vi "Intellirupter_sensor2.vi"() -> ()   [LabVIEW 2016]
uses:
  <vilib>/rvi/Emulation/niFpgaGetClockAttributes.vi
  <vilib>/rvi/Emulation/niFpgaSctlEmulationGetInTimedLoop.vi
  <vilib>/rvi/Emulation/niFpgaEmulationReportErrorSimple.vi
  <vilib>/rvi/eio/common/nirviEmuTemplateMethod_errors.vi
  <vilib>/rvi/Emulation/niFpgaCriticalErrorInLSC.vi
  <vilib>/eio/EIONode/EIONode.xnode
panel:
  out "I8 B":fxp<+/-,26,5>
  out "I8 A":fxp<+/-,26,5>
  out "V8R CA":fxp<+/-,26,5>
  out "V8R BC":fxp<+/-,26,5>
  out "V8R AB":fxp<+/-,26,5>
  out "V5R CA":fxp<+/-,26,5>
  out "V5R BC":fxp<+/-,26,5>
  out "V5R AB":fxp<+/-,26,5>
  out "I5 B":fxp<+/-,26,5>
  out "I5 A":fxp<+/-,26,5>
  out "V5L CA":fxp<+/-,26,5>
  out "V5L BC":fxp<+/-,26,5>
  out "V5L AB":fxp<+/-,26,5>
  out "V4L CA":fxp<+/-,26,5>
  out "V4L BC":fxp<+/-,26,5>
  out "V4L AB":fxp<+/-,26,5>
  out "I4 C":fxp<+/-,26,5>
  out "I4 B":fxp<+/-,26,5>
  out "I4 A":fxp<+/-,26,5>
  out "V4R CA":fxp<+/-,26,5>
  out "V4R BC":fxp<+/-,26,5>
  out "V4R AB":fxp<+/-,26,5>
  out "V2L CA":fxp<+/-,26,5>
  out "V2L BC":fxp<+/-,26,5>
  out "V2L AB":fxp<+/-,26,5>
  out "I2 C":fxp<+/-,26,5>
  out "I5 C":fxp<+/-,26,5>
  out "I2 B":fxp<+/-,26,5>
  out "I2 A":fxp<+/-,26,5>
  out "V2R CA":fxp<+/-,26,5>
  out "V2R BC":fxp<+/-,26,5>
  out "V2R AB":fxp<+/-,26,5>
  out "V7R CA":fxp<+/-,26,5>
  out "V7R BC":fxp<+/-,26,5>
  out "V7R AB":fxp<+/-,26,5>
  out "I8 C":fxp<+/-,26,5>
  out "V8L CA":fxp<+/-,26,5>
  out "V8L BC":fxp<+/-,26,5>
  out "V8L AB":fxp<+/-,26,5>
  out "I7 C":fxp<+/-,26,5>
  out "I7 B":fxp<+/-,26,5>
  out "I7 A":fxp<+/-,26,5>
  out "V7L CA":fxp<+/-,26,5>
  out "V7L BC":fxp<+/-,26,5>
  out "V7L AB":fxp<+/-,26,5>
  out "V6R CA":fxp<+/-,26,5>
  out "V6R BC":fxp<+/-,26,5>
  out "V6R AB":fxp<+/-,26,5>
  out "I6 C":fxp<+/-,26,5>
  out "I6 B":fxp<+/-,26,5>
  out "I6 A":fxp<+/-,26,5>
  out "V6L CA":fxp<+/-,26,5>
  out "V6L BC":fxp<+/-,26,5>
  out "V6L AB":fxp<+/-,26,5>
  out "V3L CA":fxp<+/-,26,5>
  out "V3L BC":fxp<+/-,26,5>
  out "V3L AB":fxp<+/-,26,5>
  out "I3 C":fxp<+/-,26,5>
  out "I3 B":fxp<+/-,26,5>
  out "I3 A":fxp<+/-,26,5>
  out "V3R CA":fxp<+/-,26,5>
  out "V3R BC":fxp<+/-,26,5>
  out "V3R AB":fxp<+/-,26,5>
  out "V1L CA":fxp<+/-,26,5>
  out "V1L BC":fxp<+/-,26,5>
  out "V1L AB":fxp<+/-,26,5>
  out "I1 C":fxp<+/-,26,5>
  out "I1 B":fxp<+/-,26,5>
  out "I1 A":fxp<+/-,26,5>
  out "V1R CA":fxp<+/-,12,5>
  out "V1R BC":fxp<+/-,26,5>
  out "V1R AB":fxp<+/-,26,5>
  in  "Count(ticks)":u32=100
  in  "Relay8":bool
  in  "Relay7":bool
  in  "Relay6":bool
  in  "Relay5":bool
  in  "Relay4":bool
  in  "Relay3":bool
  in  "Relay2":bool
  in  "Relay1":bool
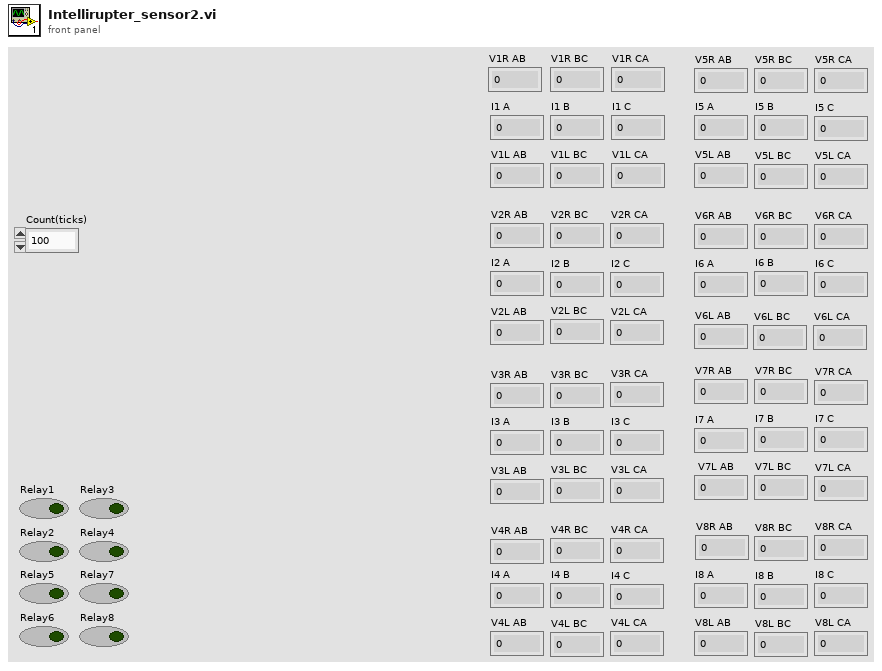
[diagram p1: front panel]
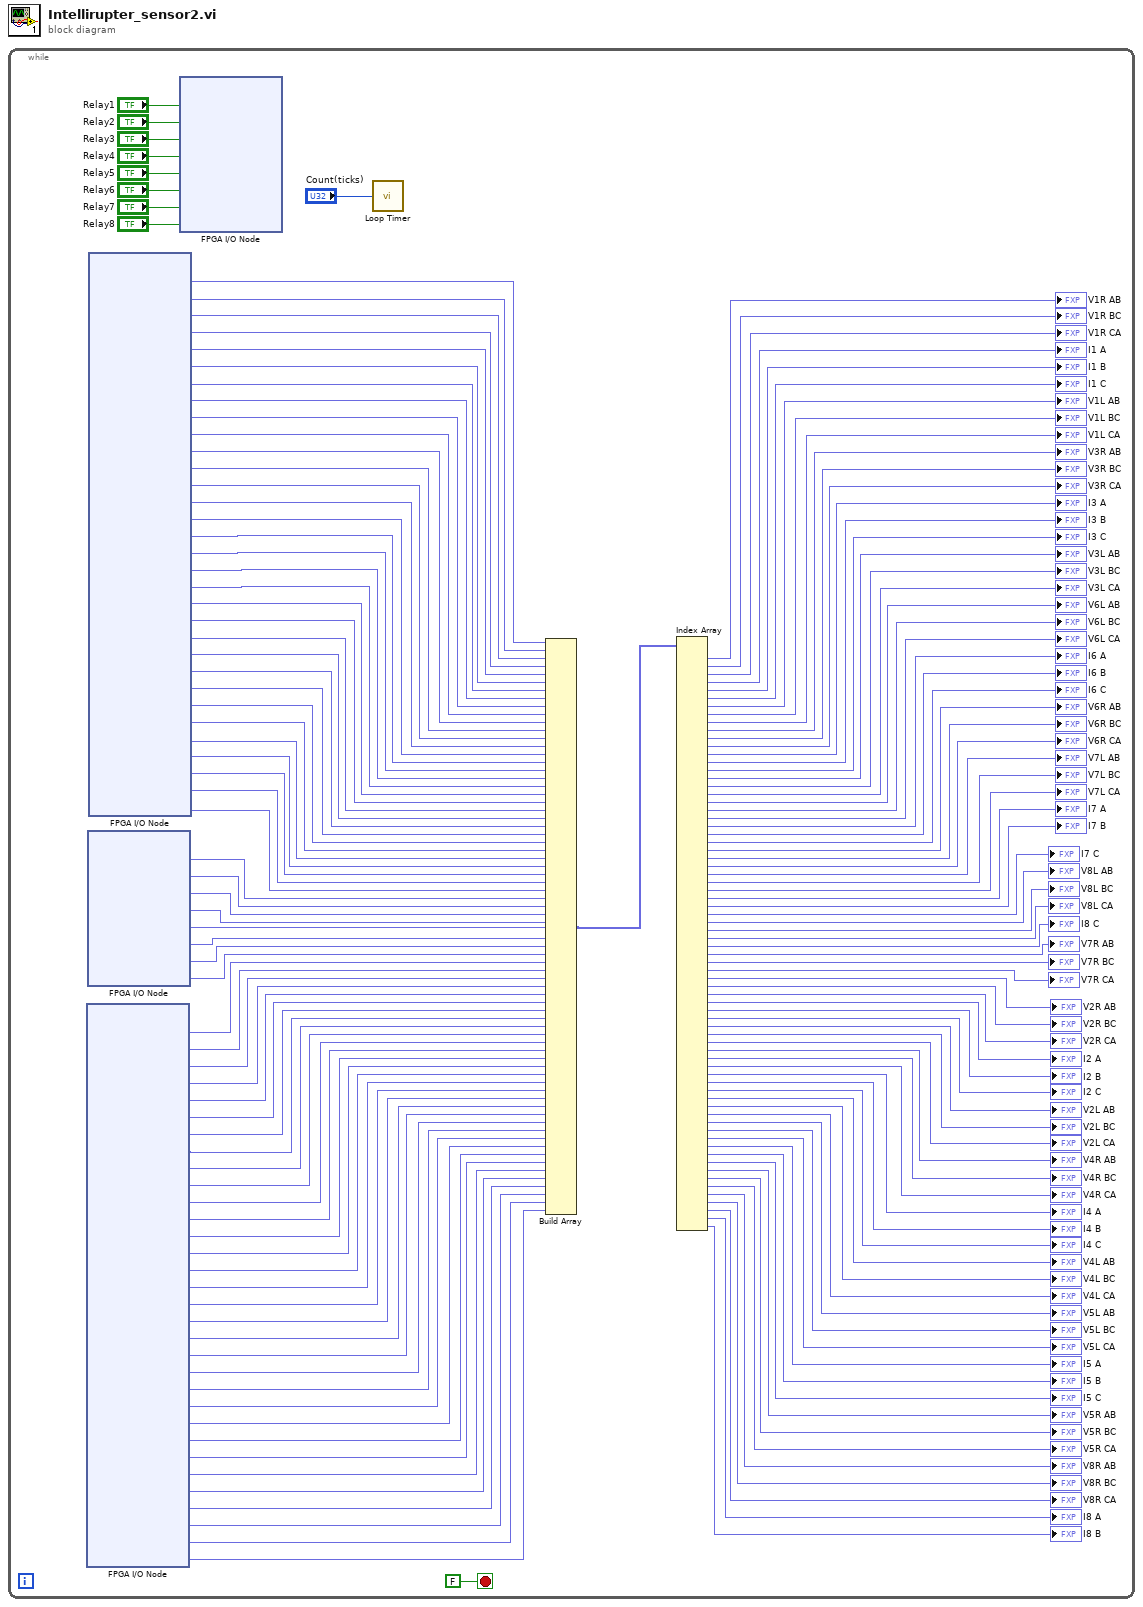
[diagram p0: block diagram]
diagram:
  n1 = while {
    stop <- FALSE stop-if-true
    n2 = xnode "FPGA I/O Node"() -> ("Mod7/AI0"=w114:fxp<+/-,26,5>, "Mod7/AI1"=w104:fxp<+/-,26,5>, "Mod7/AI2"=w103:fxp<+/-,26,5>, "Mod7/AI3"=w102:fxp<+/-,26,5>, "Mod7/AI4"=w101:fxp<+/-,26,5>, "Mod7/AI5"=w100:fxp<+/-,26,5>, "Mod7/AI6"=w99:fxp<+/-,26,5>, "Mod7/AI7"=w98:fxp<+/-,26,5>, "Mod7/AI8"=w97:fxp<+/-,26,5>, "Mod7/AI9"=w96:fxp<+/-,26,5>, "Mod7/AI10"=w95:fxp<+/-,26,5>, "Mod7/AI11"=w94:fxp<+/-,26,5>, "Mod7/AI12"=w93:fxp<+/-,26,5>, "Mod7/AI13"=w92:fxp<+/-,26,5>, "Mod7/AI14"=w74:fxp<+/-,26,5>, "Mod7/AI15"=w75:fxp<+/-,26,5>, "Mod7/AI16"=w76:fxp<+/-,26,5>, "Mod7/AI17"=w77:fxp<+/-,26,5>, "Mod7/AI18"=w78:fxp<+/-,26,5>, "Mod7/AI19"=w79:fxp<+/-,26,5>, "Mod7/AI20"=w80:fxp<+/-,26,5>, "Mod7/AI21"=w81:fxp<+/-,26,5>, "Mod7/AI22"=w82:fxp<+/-,26,5>, "Mod7/AI23"=w83:fxp<+/-,26,5>, "Mod7/AI24"=w84:fxp<+/-,26,5>, "Mod7/AI25"=w85:fxp<+/-,26,5>, "Mod7/AI26"=w86:fxp<+/-,26,5>, "Mod7/AI27"=w87:fxp<+/-,26,5>, "Mod7/AI28"=w88:fxp<+/-,26,5>, "Mod7/AI29"=w89:fxp<+/-,26,5>, "Mod7/AI30"=w90:fxp<+/-,26,5>, "Mod7/AI31"=w91:fxp<+/-,26,5>)  [unwired: 32 in, 32 out]
    n3 = xnode "FPGA I/O Node"() -> ("Mod5/AI20"=w122:fxp<+/-,26,5>, "Mod5/AI1"=w121:fxp<+/-,26,5>, "Mod5/AI2"=w120:fxp<+/-,26,5>, "Mod5/AI3"=w119:fxp<+/-,26,5>, "Mod5/AI0"=w118:fxp<+/-,26,5>, "Mod5/AI21"=w117:fxp<+/-,26,5>, "Mod5/AI22"=w116:fxp<+/-,26,5>, "Mod5/AI23"=w115:fxp<+/-,26,5>)  [unwired: 8 in, 8 out]
    n4 = xnode "FPGA I/O Node"() -> ("Mod1/AI0"=w154:fxp<+/-,26,5>, "Mod1/AI1"=w153:fxp<+/-,26,5>, "Mod1/AI2"=w152:fxp<+/-,26,5>, "Mod1/AI3"=w151:fxp<+/-,26,5>, "Mod1/AI4"=w150:fxp<+/-,26,5>, "Mod1/AI5"=w149:fxp<+/-,26,5>, "Mod1/AI6"=w148:fxp<+/-,26,5>, "Mod1/AI7"=w147:fxp<+/-,26,5>, "Mod1/AI8"=w146:fxp<+/-,26,5>, "Mod1/AI9"=w145:fxp<+/-,26,5>, "Mod1/AI10"=w144:fxp<+/-,26,5>, "Mod1/AI11"=w143:fxp<+/-,26,5>, "Mod1/AI12"=w142:fxp<+/-,26,5>, "Mod1/AI13"=w141:fxp<+/-,26,5>, "Mod1/AI14"=w140:fxp<+/-,26,5>, "Mod1/AI15"=w139:fxp<+/-,26,5>, "Mod1/AI16"=w138:fxp<+/-,26,5>, "Mod1/AI17"=w137:fxp<+/-,26,5>, "Mod1/AI18"=w136:fxp<+/-,26,5>, "Mod1/AI19"=w135:fxp<+/-,26,5>, "Mod1/AI20"=w134:fxp<+/-,26,5>, "Mod1/AI21"=w133:fxp<+/-,26,5>, "Mod1/AI22"=w132:fxp<+/-,26,5>, "Mod1/AI23"=w131:fxp<+/-,26,5>, "Mod1/AI24"=w130:fxp<+/-,26,5>, "Mod1/AI25"=w129:fxp<+/-,26,5>, "Mod1/AI26"=w128:fxp<+/-,26,5>, "Mod1/AI27"=w127:fxp<+/-,26,5>, "Mod1/AI28"=w126:fxp<+/-,26,5>, "Mod1/AI29"=w125:fxp<+/-,26,5>, "Mod1/AI30"=w124:fxp<+/-,26,5>, "Mod1/AI31"=w123:fxp<+/-,26,5>)  [unwired: 32 in, 32 out]
    n5 = xnode "FPGA I/O Node"("Mod6/DO0"="Relay1", "Mod6/DO1"="Relay2", "Mod6/DO2"="Relay3", "Mod6/DO3"="Relay4", "Mod6/DO4"="Relay5", "Mod6/DO5"="Relay6", "Mod6/DO6"="Relay7", "Mod6/DO7"="Relay8") -> ()  [unwired: 8 in, 8 out]
    n6 = call "Loop Timer"("Count(Ticks)"="Count(ticks)") -> ()  [unwired: 1 out]
    n7 = Build Array(w154, w153, w152, w151, w150, w149, w148, w147, w146, w145, w144, w143, w142, w141, w140, w139, w138, w137, w136, w135, w134, w133, w132, w131, w130, w129, w128, w127, w126, w125, w124, w123, w122, w121, w120, w119, w118, w117, w116, w115, w114, w104, w103, w102, w101, w100, w99, w98, w97, w96, w95, w94, w93, w92, w74, w75, w76, w77, w78, w79, w80, w81, w82, w83, w84, w85, w86, w87, w88, w89, w90, w91) -> (w1:fxp<+/-,26,5>[])
    n8 = Index Array(array=w1) -> (element #1=→"V1R AB":fxp<+/-,26,5>, element #2=→"V1R BC":fxp<+/-,26,5>, element #3=→"V1R CA":fxp<+/-,26,5>, element #4=→"I1 A":fxp<+/-,26,5>, element #5=→"I1 B":fxp<+/-,26,5>, element #6=→"I1 C":fxp<+/-,26,5>, element #7=→"V1L AB":fxp<+/-,26,5>, element #8=→"V1L BC":fxp<+/-,26,5>, element #9=→"V1L CA":fxp<+/-,26,5>, element #10=→"V3R AB":fxp<+/-,26,5>, element #11=→"V3R BC":fxp<+/-,26,5>, element #12=→"V3R CA":fxp<+/-,26,5>, element #13=→"I3 A":fxp<+/-,26,5>, element #14=→"I3 B":fxp<+/-,26,5>, element #15=→"I3 C":fxp<+/-,26,5>, element #16=→"V3L AB":fxp<+/-,26,5>, element #17=→"V3L BC":fxp<+/-,26,5>, element #18=→"V3L CA":fxp<+/-,26,5>, element #19=→"V6L AB":fxp<+/-,26,5>, element #20=→"V6L BC":fxp<+/-,26,5>, element #21=→"V6L CA":fxp<+/-,26,5>, element #22=→"I6 A":fxp<+/-,26,5>, element #23=→"I6 B":fxp<+/-,26,5>, element #24=→"I6 C":fxp<+/-,26,5>, element #25=→"V6R AB":fxp<+/-,26,5>, element #26=→"V6R BC":fxp<+/-,26,5>, element #27=→"V6R CA":fxp<+/-,26,5>, element #28=→"V7L AB":fxp<+/-,26,5>, element #29=→"V7L BC":fxp<+/-,26,5>, element #30=→"V7L CA":fxp<+/-,26,5>, element #31=→"I7 A":fxp<+/-,26,5>, element #32=→"I7 B":fxp<+/-,26,5>, element #33=→"I7 C":fxp<+/-,26,5>, element #34=→"V8L AB":fxp<+/-,26,5>, element #35=→"V8L BC":fxp<+/-,26,5>, element #36=→"V8L CA":fxp<+/-,26,5>, element #37=→"I8 C":fxp<+/-,26,5>, element #38=→"V7R AB":fxp<+/-,26,5>, element #39=→"V7R BC":fxp<+/-,26,5>, element #40=→"V7R CA":fxp<+/-,26,5>, element #41=→"V2R AB":fxp<+/-,26,5>, element #42=→"V2R BC":fxp<+/-,26,5>, element #43=→"V2R CA":fxp<+/-,26,5>, element #44=→"I2 A":fxp<+/-,26,5>, element #45=→"I2 B":fxp<+/-,26,5>, element #46=→"I2 C":fxp<+/-,26,5>, element #47=→"V2L AB":fxp<+/-,26,5>, element #48=→"V2L BC":fxp<+/-,26,5>, element #49=→"V2L CA":fxp<+/-,26,5>, element #50=→"V4R AB":fxp<+/-,26,5>, element #51=→"V4R BC":fxp<+/-,26,5>, element #52=→"V4R CA":fxp<+/-,26,5>, element #53=→"I4 A":fxp<+/-,26,5>, element #54=→"I4 B":fxp<+/-,26,5>, element #55=→"I4 C":fxp<+/-,26,5>, element #56=→"V4L AB":fxp<+/-,26,5>, element #57=→"V4L BC":fxp<+/-,26,5>, element #58=→"V4L CA":fxp<+/-,26,5>, element #59=→"V5L AB":fxp<+/-,26,5>, element #60=→"V5L BC":fxp<+/-,26,5>, element #61=→"V5L CA":fxp<+/-,26,5>, element #62=→"I5 A":fxp<+/-,26,5>, element #63=→"I5 B":fxp<+/-,26,5>, element #64=→"I5 C":fxp<+/-,26,5>, element #65=→"V5R AB":fxp<+/-,26,5>, element #66=→"V5R BC":fxp<+/-,26,5>, element #67=→"V5R CA":fxp<+/-,26,5>, element #68=→"V8R AB":fxp<+/-,26,5>, element #69=→"V8R BC":fxp<+/-,26,5>, element #70=→"V8R CA":fxp<+/-,26,5>, element #71=→"I8 A":fxp<+/-,26,5>, element #72=→"I8 B":fxp<+/-,26,5>)  [unwired: 72 in]
  }
